vi "TDCcalibration.vi"(7 "TDC offset":u32 format="%x", 8 "error in (no error)":errorcluster, 9 "ChipID":u32=65535 format="%x", 10 "LayerID":u32=65535 format="%x", 11 "connection ID":refnum<k5>) -> (0 "error out":errorcluster, 2 "TDC calibration data":u32[](array[numeric]) format="%x", 3 "connection ID out":refnum<k5>, 4 "Answer":string)   [LabVIEW 2015, in "VIPM2.lvlib"]
uses:
  VIPM2.lvlib
panel:
  out "Ready to receive parameters":string
  # "TDC Calibration"
  # "Time to Digital Conversion"
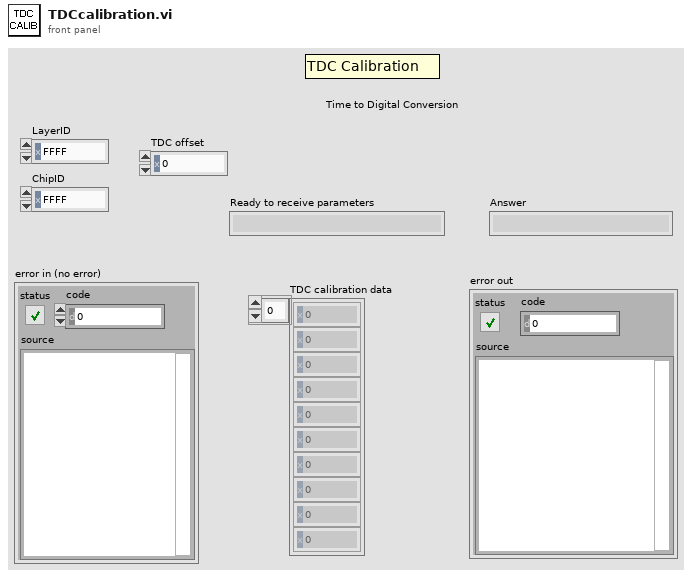
[diagram p1: front panel]
types:
  T1 = enum16{"Standard", "Buffered", "CRLF", "Immediate"}
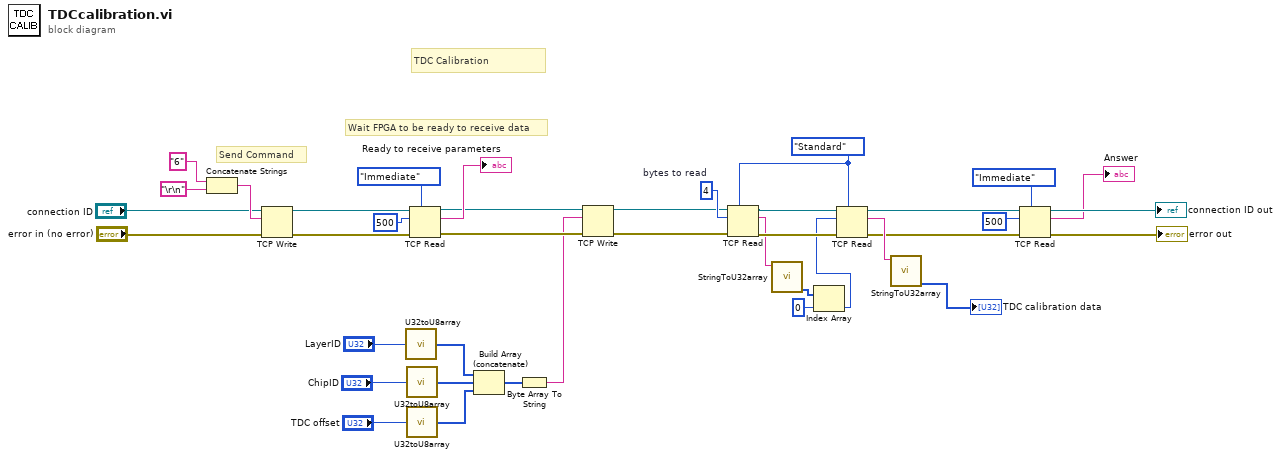
[diagram p0: block diagram]
diagram:
  w11 = 4  # bytes to read
  w12 = T1."Standard" ("mode (standard)")
  # "Wait FPGA to be ready to receive data"
  # "Send Command"
  # "TDC Calibration"
  n1 = Concatenate Strings("6" ("string"), "\r\n") -> (w37:string)
  n2 = TCP Write(connection ID="connection ID", data in=w37, error in (no error)="error in (no error)") -> (connection ID out=w31:refnum<k5>, error out=w30:errorcluster)  [unwired: 1 in, 1 out]
  n3 = call "U32toU8array.vi"("x"="LayerID") -> ("ArrayU8"=w19:u8[])
  n4 = call "U32toU8array.vi"("x"="ChipID") -> ("ArrayU8"=w17:u8[])
  n5 = call "U32toU8array.vi"("x"="TDC offset") -> ("ArrayU8"=w1:u8[])
  n6 = TCP Read(connection ID=w31, bytes to read=500, error in (no error)=w30, 7:T1."Immediate" ("mode (standard)")) -> (connection ID out=w28:refnum<k5>, data out=→"Ready to receive parameters":string, error out=w27:errorcluster)  [unwired: 1 in]
  n7 = Build Array (concatenate)(w19, w17, w1) -> (w20:u8[])
  n8 = Byte Array To String(unsigned byte array=w20) -> (string=w26:string)
  n9 = TCP Write(connection ID=w28, data in=w26, error in (no error)=w27) -> (connection ID out=w7:refnum<k5>, error out=w6:errorcluster)  [unwired: 1 in, 1 out]
  n10 = TCP Read(connection ID=w7, bytes to read=w11, error in (no error)=w6, 7:w12) -> (connection ID out=w16:refnum<k5>, data out=w10:string, error out=w15:errorcluster)  [unwired: 1 in]
  n11 = call "StringToU32array.vi"("String"=w10) -> ("U32array"=w9:u32[])  [unwired: 2 out]
  n12 = Index Array(array=w9, index=0) -> (element=w13:u32)
  n13 = TCP Read(connection ID=w16, bytes to read=w13, error in (no error)=w15, 7:w12) -> (connection ID out=w5:refnum<k5>, data out=w8:string, error out=w4:errorcluster)  [unwired: 1 in]
  n14 = call "StringToU32array.vi"("String"=w8) -> ("U32array"=→"TDC calibration data":u32[])  [unwired: 2 out]
  n15 = TCP Read(connection ID=w5, bytes to read=500, error in (no error)=w4, 7:T1."Immediate" ("mode (standard)")) -> (connection ID out=→"connection ID out":refnum<k5>, data out=→"Answer":string, error out=→"error out":errorcluster)  [unwired: 1 in]
